vi "CloseVISA.vi"(8 "error in (no error)":errorcluster, 11 "ConfocalStage in":refnum<class "ConfocalStage.lvclass">) -> (0 "error out":errorcluster, 3 "ConfocalStage out":refnum<class "ConfocalStage.lvclass">)   [LabVIEW 2012, in "ConfocalStage.lvclass"]
uses:
  ConfocalStage.lvclass
  ConfocalStage.lvclass/ConfocalStage.ctl
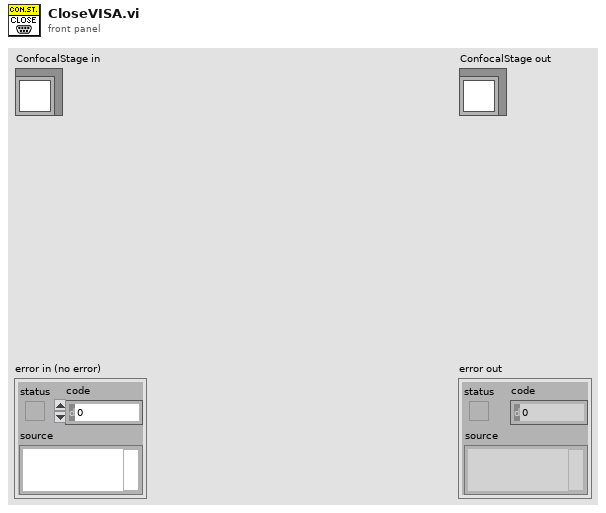
[diagram p1: front panel]
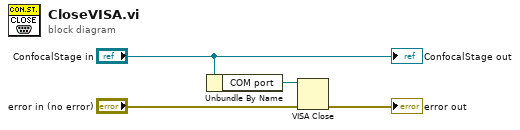
[diagram p0: block diagram]
diagram:
  n1 = Unbundle By Name("ConfocalStage in") -> ("COM port"=w1:refnum<visa-resource-name>)
  n2 = VISA Close(VISA resource name=w1, error in (no error)="error in (no error)") -> (error out=→"error out":errorcluster)
  "ConfocalStage out" <- "ConfocalStage in"
